vi "Create Retention Policy.vi"(0 "InfluxDB in":refnum<class "Client.lvclass">, 5 "Database name":string, 11 "error in (no error)":errorcluster) -> (4 "InfluxDB out":refnum<class "Client.lvclass">, 15 "error out":errorcluster)   [LabVIEW 2018, in "InfluxDB Client.lvlib" / "Client.lvclass"]
doc: "Creates a database."
uses:
  Client.lvclass
panel:
  in  "IsDefault":bool
  in  "ReplicaN":i32 format="%<%H:%M:%S>t"
  in  "Duration":i32 format="%<%H:%M:%S>t"
  in  "Retention policy name":string
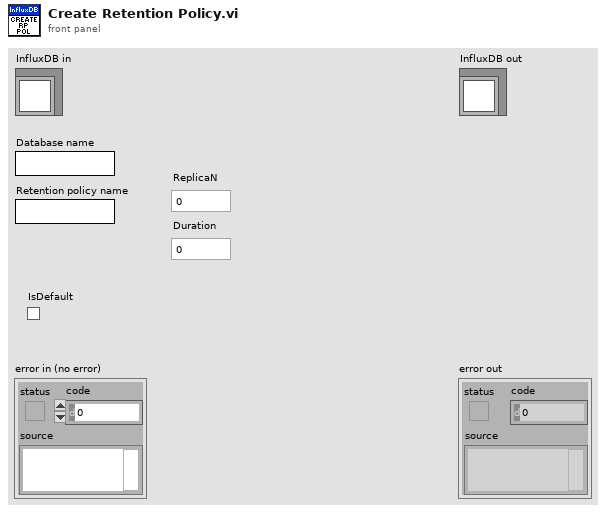
[diagram p1: front panel]
types:
  T1 = typedef "Dictionary Object RefNum__ogtk.ctl" = refnum<k1>
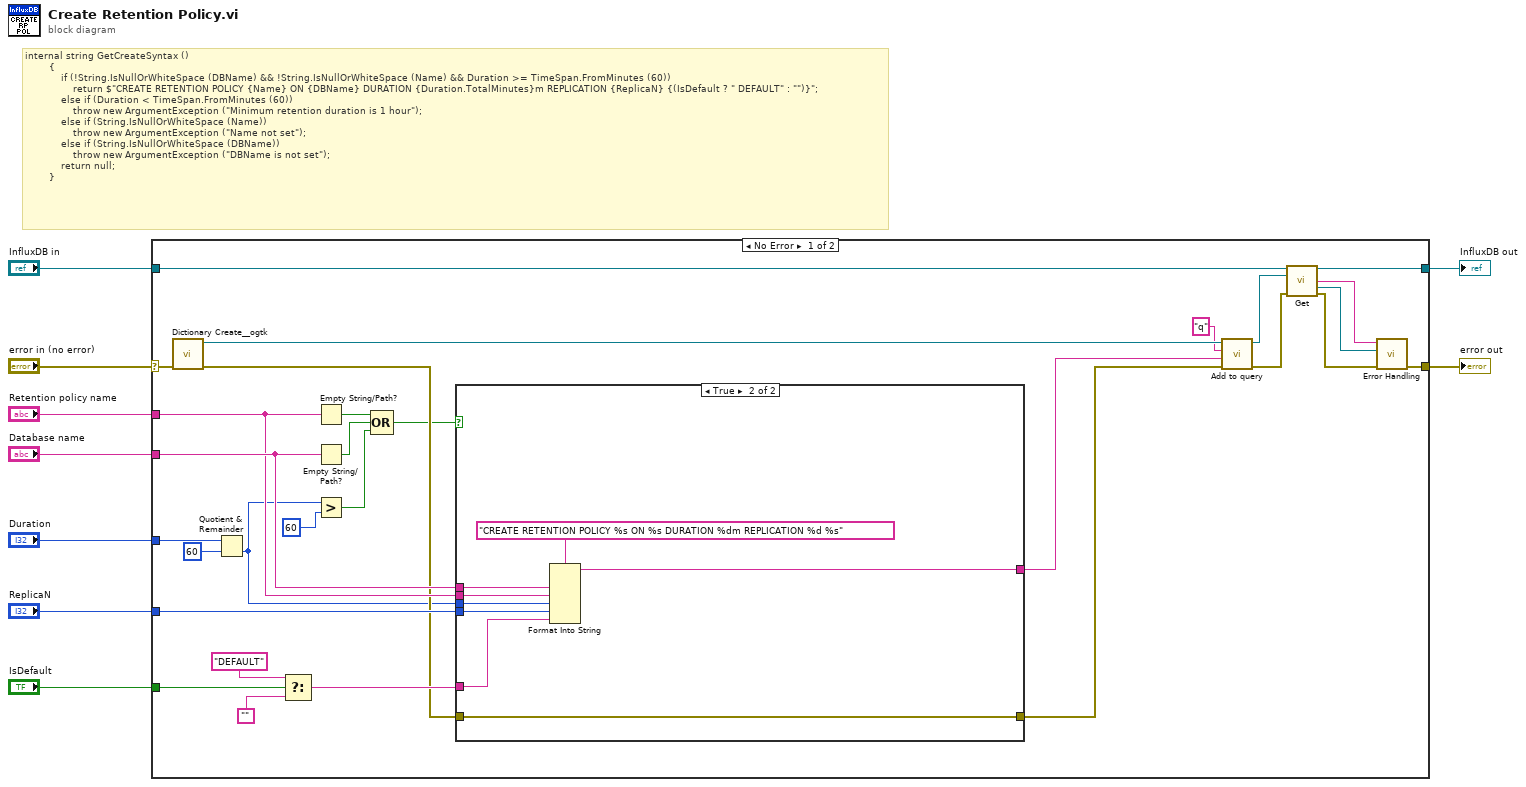
[diagram p0: block diagram]
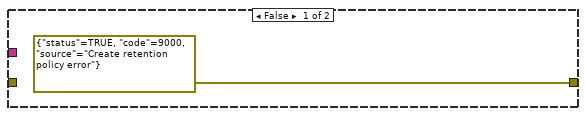
[diagram p2: hidden frame]
diagram:
  # "internal string GetCreateSyntax ()\n        {\n            if (!String.IsNullOrWhiteSpace (DBName) && !String.IsNullOrWhiteSpace (Name) && Duration >= TimeSpan.FromMinutes (60))\n                return $\"CREATE RETENTION POLICY {Name} ON {DBName} DURATION {Duration.TotalMinutes}m REPLICATION {ReplicaN} {(IsDefault ? \" DEFAULT\" : \"\")}\";\n            else if (Duration < TimeSpan.FromMinutes (60))\n                throw new ArgumentException (\"Minimum retention duration is 1 hour\");\n            else if (String.IsNullOrWhiteSpace (Name))\n                throw new ArgumentException (\"Name not set\");\n            else if (String.IsNullOrWhiteSpace (DBName))\n                throw new ArgumentException (\"DBName is not set\");\n            return null;\n        }"
  n1 = case shown="No Error" "error in (no error)" {
    selector: "error in (no error)" -> [w25 w49]
    tunnel: [w31 w49] -> w9
    tunnel: [w37 w48] -> w7
    tunnel: "InfluxDB in" -> [w38 w48]
    tunnel: "Database name" -> [w23 _]
    tunnel: "Retention policy name" -> [w22 _]
    tunnel: "Duration" -> [w24 _]
    tunnel: "ReplicaN" -> [w21 _]
    tunnel: "IsDefault" -> [w20 _]
    frame No Error {
      n2 = call <userlib>:"Dictionary Create__ogtk.vi"("error in (no error)"=w25) -> ("error out"=w15:errorcluster, "dictionary out"=w36:T1)  [unwired: 9 in]
      n3 = Quotient & Remainder(x=w24, y=60) -> (floor(x/y)=w12:i32)  [unwired: 1 out]
      n4 = Select(t="DEFAULT" ("format string"), s=w20, f="") -> (s? t:f=w17:string)
      n5 = Empty String/Path?(string/path=w22) -> (empty?=w27:bool)
      n6 = Empty String/Path?(string/path=w23) -> (empty?=w28:bool)
      n7 = Greater?(x=w12, y=60) -> (0:w10:bool)
      n8 = Compound Arithmetic op=OR(w27, w28, w10) -> (w13:bool)
      n9 = case shown="True" w13 {
        tunnel: w23 -> [_ w46]
        tunnel: w22 -> [_ w45]
        tunnel: w12 -> [_ w44]
        tunnel: w21 -> [_ w43]
        tunnel: w17 -> [_ w42]
        tunnel: [_ w41] -> w16
        tunnel: w15 -> [_ w40]
        tunnel: [errorcluster {"status"=TRUE, "code"=9000, "source"="Create retention policy error"} ("error constant") w40] -> w14
        frame False {
        }
        frame True {
          n10 = Format Into String(format string="CREATE RETENTION POLICY %s ON %s DURATION %dm REPLICATION %d %s", w46, w45, w44, w43, w42) -> (resulting string=w41:string)  [unwired: 2 in, 1 out]
        }
      }
      n11 = call "Add to query.vi"("error in (no error)"=w14, "Value"=w16, "Parameter"="q" ("String"), "Query in"=w36) -> ("error out"=w33:errorcluster, "Query out"=w34:T1)  [unwired: 6 in]
      n12 = call "Get.vi"("InfluxDB Client in"=w38, "Query"=w34, "error in (no error)"=w33) -> ("InfluxDB Client out"=w37:refnum<class "Client.lvclass">, "Status code"=w30:string, "Headers"=w29:T1, "error out"=w32:errorcluster)  [unwired: 8 in, 1 out]
      n13 = call "Error Handling.vi"("error in (no error)"=w32, "HTTP headers"=w29, "HTTP status code"=w30) -> ("error out"=w31:errorcluster)  [unwired: 8 in]
    }
    frame Error {
    }
  }
  "error out" <- w9
  "InfluxDB out" <- w7
